vi "Launch Wizard.vi"(8 "error in (no error)":errorcluster, 10 "Controller in":refnum<class "Controller.lvclass">, 11 "New Project Wizard in":refnum<class "Update Project Wizard.lvclass">) -> (0 "error out":errorcluster, 3 "Caller-To-Actor Enqueuer":refnum<class "Message Enqueuer.lvclass">)   [LabVIEW 2013, in "SET Project Editor.lvlib" / "Update Project Wizard.lvclass"]
uses:
  Update Project Wizard.lvclass
  <vilib>/ActorFramework/Message Enqueuer/Message Enqueuer.lvclass
  Controller/Controller.lvclass
  Controller/Controller.lvclass/Controller.ctl
  Update Project Wizard.lvclass/Update Project Wizard.ctl
  UI Wizard/UI Wizard.lvclass
  Controller/Read Default Path.vi
  SET Project Data/Project Data Class/Project Data.lvclass
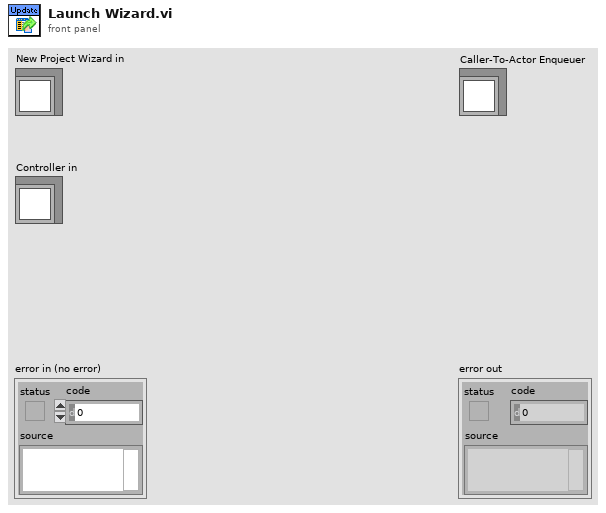
[diagram p1: front panel]
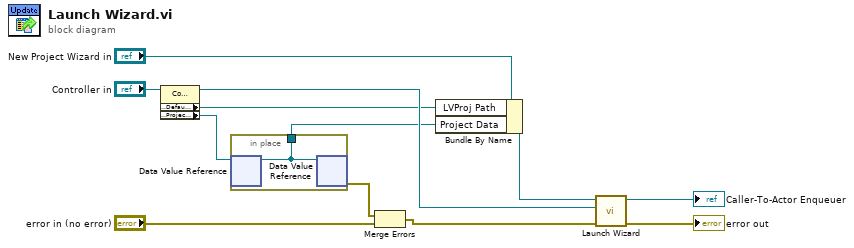
[diagram p0: block diagram]
diagram:
  n1 = property class="Controller.lvclass"(reference="Controller in") -> (reference out=w9:refnum<class "Controller.lvclass">, "Properties:Default Path"=w6:path, "Properties:Project Data ref"=w5:refnum<data-value>)  [unwired: 1 in, 1 out]
  n2 = in-place {
    in-place-border: [w13] -> w4
    n3 = in-place-dvr #1(w5) -> (w13:refnum<class "Project Data.lvclass">)  [unwired: 1 out]
    n4 = in-place-dvr #1(w13) -> (w2:errorcluster)  [unwired: 1 out]
  }
  n5 = Merge Errors(w2, "error in (no error)") -> (w1:errorcluster)
  n6 = Bundle By Name(cluster="New Project Wizard in", "LVProj Path"=w6, "Project Data"=w4) -> (w7:refnum<class "Update Project Wizard.lvclass">)
  n7 = call-parent "Launch Wizard.vi"("error in (no error)"=w1, "Controller in"=w9, "UI Wizard in"=w7) -> ("error out"=→"error out":errorcluster, "Caller-To-Actor Enqueuer"=→"Caller-To-Actor Enqueuer":refnum<class "Message Enqueuer.lvclass">)  [unwired: 7 in]
